vi "Decrement.vi"(11 "x":dbl) -> (3 "x-1":dbl)   [LabVIEW 2014]
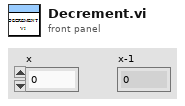
[diagram p1: front panel]
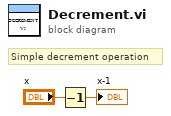
[diagram p0: block diagram]
diagram:
  # "Simple decrement operation"
  n1 = Decrement(x="x") -> (x-1=→"x-1":dbl)
